vi "_API_BINANCE_GET_USDT_FUTURES_leverage.vi"(0 "BinanceAPI in":refnum<class "BinanceAPI_.lvclass">, 5 "leverage":cluster{"Symbol (eg. BTCUSDT)":string}, 11 "error in (no error)":errorcluster) -> (4 "BinanceAPI out":refnum<class "BinanceAPI_.lvclass">, 6 "Leverage numeric":dbl format="%#.6f", 14 "Leverage string":string, 15 "error out":errorcluster)   [LabVIEW 2022 SP3, in "BinanceAPI_.lvclass"]
doc: "Levereage used in pair of crypto form future account"
uses:
  BinanceAPI_.lvclass
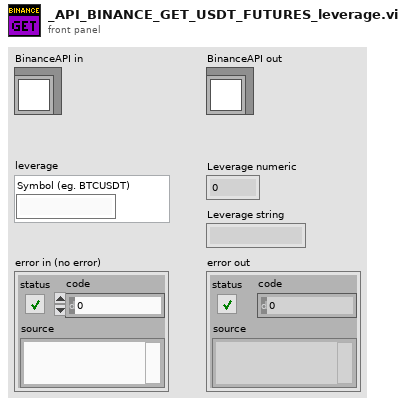
[diagram p1: front panel]
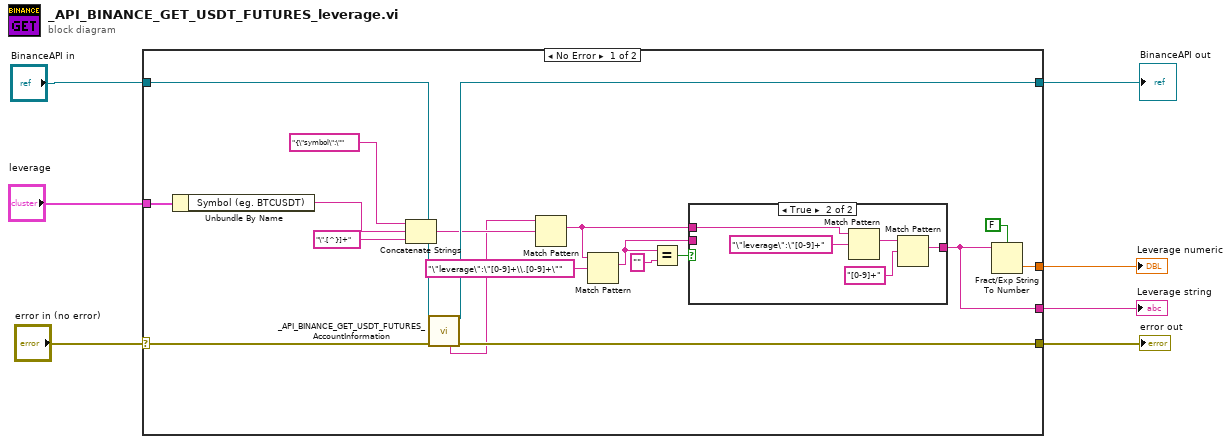
[diagram p0: block diagram]
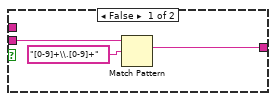
[diagram p2: hidden frame]
diagram:
  n1 = case shown="No Error" "error in (no error)" {
    selector: "error in (no error)" -> [w10 w34]
    tunnel: [w23 _] -> w7
    tunnel: [w21 _] -> w6
    tunnel: [w18 w34] -> w5
    tunnel: [w17 w35] -> w1
    tunnel: "BinanceAPI in" -> [w16 w35]
    tunnel: "leverage" -> [w9 _]
    frame No Error {
      n2 = Unbundle By Name(w9) -> ("Symbol (eg. BTCUSDT)"=w8:string)
      n3 = Concatenate Strings("{\"symbol\":\"" ("regular expression"), w8, "\".[^}]+" ("string")) -> (w13:string)
      n4 = call "_API_BINANCE_GET_USDT_FUTURES_AccountInformation.vi"("BinanceAPI in"=w16, "error in (no error)"=w10) -> ("BinanceAPI out"=w17:refnum<class "BinanceAPI_.lvclass">, "Data"=w12:string, "error out"=w18:errorcluster)  [unwired: 10 in, 1 out]
      n5 = Match Pattern(string=w12, regular expression=w13) -> (match substring=w11:string)  [unwired: 1 in, 3 out]
      n6 = Match Pattern(string=w11, regular expression="\"leverage\":\"[0-9]+\\.[0-9]+\"") -> (match substring=w20:string)  [unwired: 1 in, 3 out]
      n7 = Equal?(x=w20, y="" ("match substring")) -> (x = y?=w19:bool)
      n8 = case shown="True" w19 {
        tunnel: [w27 w30] -> w21
        tunnel: w20 -> [w26 _]
        tunnel: w11 -> [_ w32]
        frame False {
          n9 = Match Pattern(string=w26, regular expression="[0-9]+\\.[0-9]+") -> (match substring=w27:string)  [unwired: 1 in, 3 out]
        }
        frame True {
          n10 = Match Pattern(string=w32, regular expression="\"leverage\":\"[0-9]+") -> (match substring=w29:string)  [unwired: 1 in, 3 out]
          n11 = Match Pattern(string=w29, regular expression="[0-9]+") -> (match substring=w30:string)  [unwired: 1 in, 3 out]
        }
      }
      n12 = Fract/Exp String To Number(use system decimal point (T)=FALSE, string=w21) -> (number=w23:dbl)  [unwired: 2 in, 1 out]
    }
    frame Error {
    }
  }
  "Leverage numeric" <- w7
  "Leverage string" <- w6
  "error out" <- w5
  "BinanceAPI out" <- w1
